vi "FullSetup.vi"() -> ()   [LabVIEW 2020]
uses:
  <vilib>/MakerHub/LINX/Private/Device/Type Defs/Stimulus Pulse.ctl
  <vilib>/MakerHub/LINX/Public/Peripherals/Analog/Analog Read 1 Chan.vi
  <vilib>/MakerHub/LINX/Public/Peripherals/Digital/Digital Write 1 Chan.vi
  <vilib>/MakerHub/LINX/Public/Peripherals/PWM/PWM Set Duty Cycle 1 Chan.vi
  <vilib>/MakerHub/LINX/Public/Peripherals/Analog/Analog Read N Chans.vi
  <vilib>/MakerHub/LINX/Public/Peripherals/Digital/Digital Write N Chans.vi
  <vilib>/MakerHub/LINX/Private/Local IO/LinxAnalogRead.vi
  <vilib>/MakerHub/LINX/Public/Utilities/Check Channel.vi
  <vilib>/MakerHub/LINX/Private/Local IO/LinxDigitalWrite.vi
  <vilib>/MakerHub/LINX/Public/Utilities/Open Serial.vi
  <vilib>/MakerHub/LINX/Private/Utilties/Generate Error.vi
  <vilib>/MakerHub/LINX/Public/Peripherals/PWM/PWM Set Duty Cycle N Chans.vi
  <vilib>/MakerHub/LINX/LMH-LINX.lvlib
  <vilib>/MakerHub/LINX/Private/Device/Device.lvlib
panel:
  out "Light Intensity":dbl
  out "Count Inside room":i32
  out "Distance OUT":dbl
  out "Waveform Chart 3":dbl(graph)
  in  "DO Channel OUT":u8
  in  "DI Channel OUT":u8
  out "Distance IN":dbl
  out "Waveform Chart":dbl(graph)
  in  "DO Channel IN":u8
  in  "DI Channe INl":u8
  in  "stop":bool
  out "Temperature":dbl
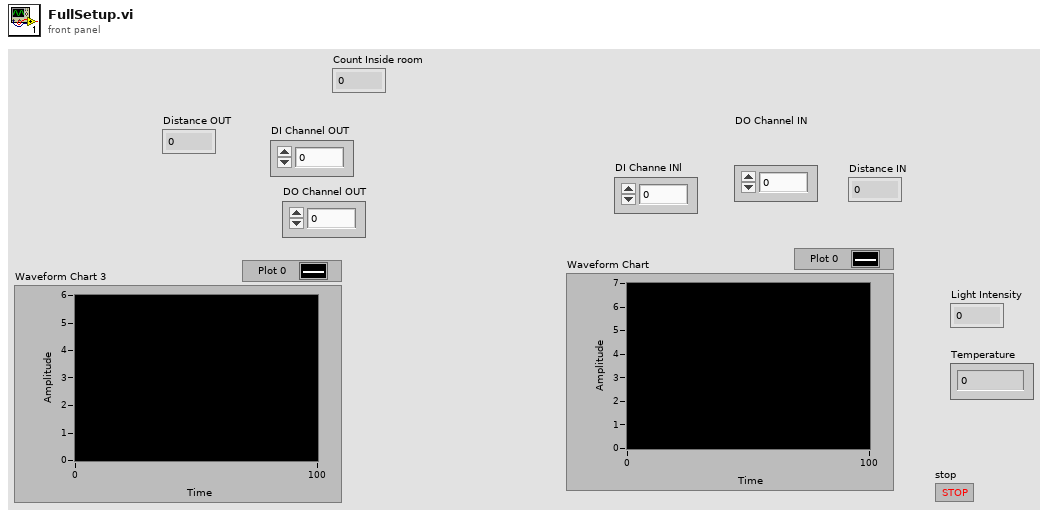
[diagram p1: front panel]
types:
  T1 = typedef "LMH-LINX.lvlib/LINX Ref.ctl" = cluster{"IO":T2, "Interface":T3, "LINX Device Config":T4}
  T2 = typedef "LMH-LINX.lvlib/Platform.ctl" = enum16{"Remote", "Local"}
  T3 = typedef "LMH-LINX.lvlib/Interface.ctl" = enum16{"Serial", "TCP"}
  T4 = typedef "LMH-LINX.lvlib/Device.lvlib/LINX Device Config.ctl" = cluster{"Interface":T3, "COM Port":refnum<visa-resource-name>, "TCP Configuration":T5, "Device Family":u8, "Device ID":u8, "Device Name":string, "TCP Ref":refnum<k5>, "Channels":T6}
  T5 = typedef "LMH-LINX.lvlib/Device.lvlib/TCP Config.ctl" = cluster{"IP Address":string, "Port":u16}
  T6 = typedef "LMH-LINX.lvlib/Channels.ctl" = cluster{"DI":u8[], "DO":u8[], "AI":u8[], "AO":u8[], "PWM":u8[], "QE":u8[], "UART":u8[], "I2C 2":u8[], "SPI":u8[], "CAN":u8[], "Servo":u8[], "AI Ref (V)":dbl, "AI Resolution (Bits)":u8, "AO Ref (V)":dbl, "AO Resolution (Bits)":u8}
  T7 = typedef "LMH-LINX.lvlib/Device.lvlib/Stimulus Pulse.ctl" = enum16{"None", "Active Low", "Active High"}
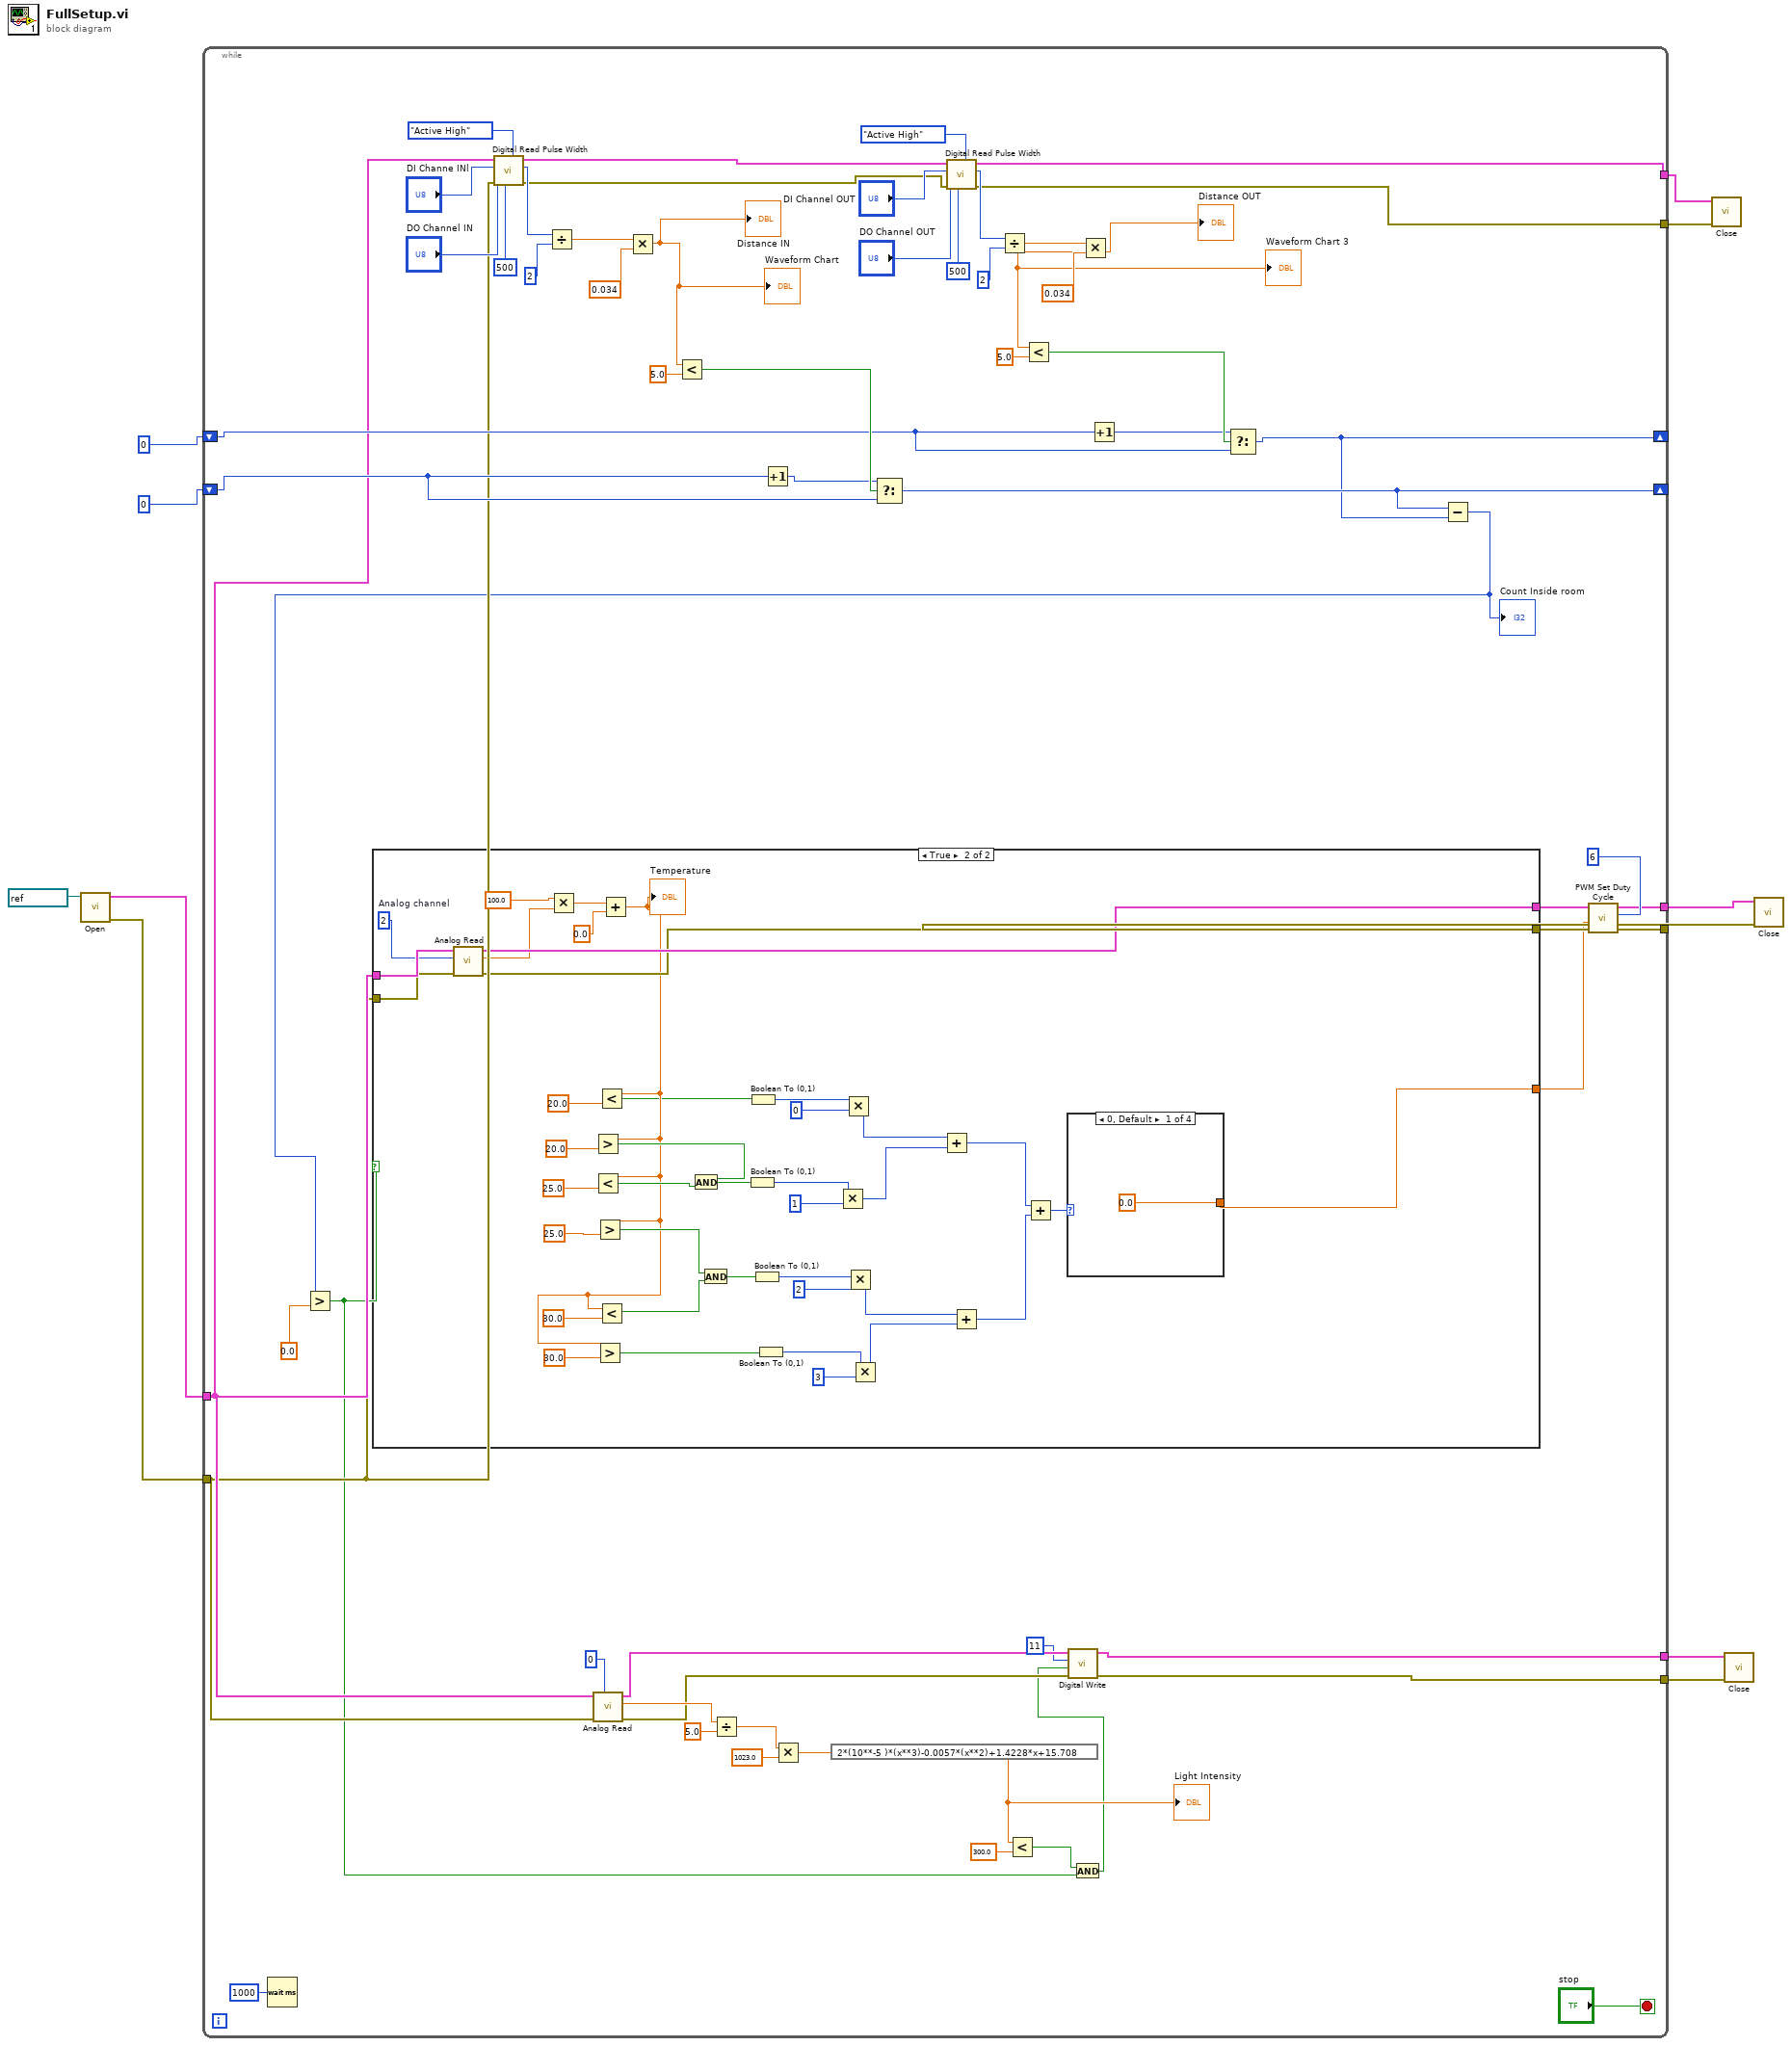
[diagram p0: block diagram]
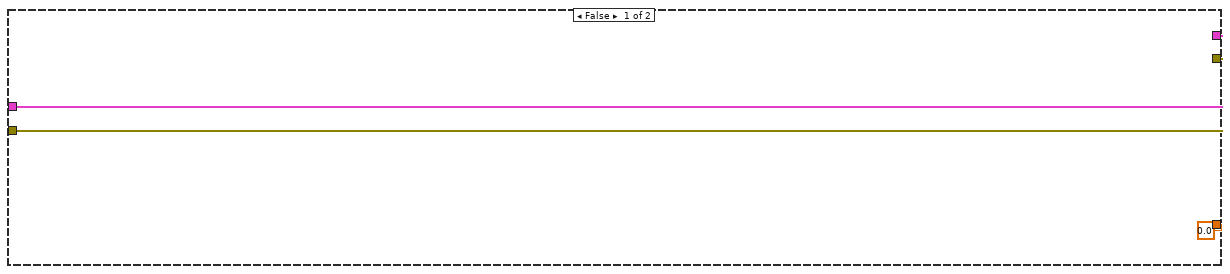
[diagram p2: hidden frame]
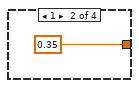
[diagram p3: hidden frame]
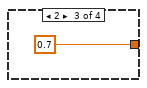
[diagram p4: hidden frame]
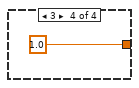
[diagram p5: hidden frame]
diagram:
  n1 = call-poly <vilib>:"Open.vi"("Serial Port"=refnum<visa-resource-name> "COM4") -> ("Error Out"=w9:errorcluster, "LINX Resource"=w11:T1)  [unwired: 8 in, 1 out]
  n2 = while {
    tunnel: w11 -> [w21]
    tunnel: [w66] -> w10
    tunnel: w9 -> [w20]
    tunnel: [w64] -> w8
    tunnel: [w38] -> w6
    shift-right: [w34] -> _
    shift-left: 0 -> [w37]
    shift-right: [w35] -> _
    shift-left: 0 -> [w36]
    tunnel: [w33] -> w3
    tunnel: [w18] -> w2
    tunnel: [w17] -> w1
    stop <- "stop" stop-if-true
    n3 = Wait (ms)(milliseconds to wait=u32 1000) -> ()  [unwired: 1 out]
    n4 = call <vilib>:"Digital Read Pulse Width.vi"("Stimulus Pulse (Active High)"=Stimulus_Pulse."Active High", "Timeout  (250 mS)"=u32 500, "Error In"=w20, "DO Channel"="DO Channel IN", "DI Channel"="DI Channe INl", "LINX Resource"=w21) -> ("Error Out"=w32:errorcluster, "Pulse Width (uS)"=w61:u32, "LINX Resource"=w47:T1)  [unwired: 3 in]
    n5 = Divide(x=w61, y=2) -> (x/y=w59:dbl)
    n6 = call-poly <vilib>:"Analog Read.vi"("Analog Ref Override (V)"=0, "Error In"=w20, "LINX Resource"=w21) -> ("Error Out"=w19:errorcluster, "Voltage"=w29:dbl, "LINX Resource"=w25:T1)  [unwired: 5 in, 1 out]
    n7 = Multiply(x=w59, y=0.034) -> (x*y=w46:dbl)
    "Waveform Chart" <- w46
    "Distance IN" <- w46
    n8 = Less?(x=w46, y=5.0) -> (x < y?=w42:bool)
    n9 = Divide(x=w29, y=5.0) -> (x/y=w27:dbl)
    n10 = Increment(x=w36) -> (x+1=w41:i32)
    n11 = Multiply(x=w27, y=1023.0) -> (x*y=w26:dbl)
    n12 = expression code="2*(10**-5 )*(x**3)-0.0057*(x**2)+1.4228*x+15.708"(w26) -> (w23:dbl)
    "Light Intensity" <- w23
    n13 = Select(t=w41, s=w42, f=w36) -> (s? t:f=w35:i32)
    n14 = call <vilib>:"Digital Read Pulse Width.vi"("Stimulus Pulse (Active High)"=Stimulus_Pulse."Active High", "Timeout  (250 mS)"=u32 500, "Error In"=w32, "DO Channel"="DO Channel OUT", "DI Channel"="DI Channel OUT", "LINX Resource"=w47) -> ("Error Out"=w33:errorcluster, "Pulse Width (uS)"=w53:u32, "LINX Resource"=w38:T1)  [unwired: 3 in]
    n15 = Divide(x=w53, y=2) -> (x/y=w51:dbl)
    n16 = Less?(x=w23, y=300.0) -> (x < y?=w15:bool)
    n17 = Multiply(x=w51, y=0.034) -> (x*y=w43:dbl)
    "Waveform Chart 3" <- w43
    "Distance OUT" <- w43
    n18 = Less?(x=w43, y=5.0) -> (x < y?=w40:bool)
    n19 = Increment(x=w37) -> (x+1=w39:i32)
    n20 = Select(t=w39, s=w40, f=w37) -> (s? t:f=w34:i32)
    n21 = Subtract(x=w35, y=w34) -> (x-y=w16:i32)
    "Count Inside room" <- w16
    n22 = Greater?(x=w16, y=0.0) -> (0:w13:bool)
    n23 = case shown="True" w13 {
      tunnel: w21 -> [w73 w114]
      tunnel: [w73 w113] -> w67
      tunnel: [w72 w112] -> w65
      tunnel: [0.0 w80] -> w70
      tunnel: w20 -> [w72 w75]
      frame False {
      }
      frame True {
        w111 = 2  # Analog channel
        n24 = call-poly <vilib>:"Analog Read.vi"("Error In"=w75, "Analog Channel"=w111, "LINX Resource"=w114) -> ("Error Out"=w112:errorcluster, "Voltage"=w109:dbl, "LINX Resource"=w113:T1)  [unwired: 5 in, 1 out]
        n25 = Multiply(x=100.0, y=w109) -> (x*y=w107:dbl)
        n26 = Add(x=w107, y=0.0) -> (x+y=w88:dbl)
        "Temperature" <- w88
        n27 = Greater?(x=w88, y=20.0) -> (0:w100:bool)
        n28 = Less?(x=w88, y=25.0) -> (x < y?=w99:bool)
        n29 = Greater?(x=w88, y=25.0) -> (0:w93:bool)
        n30 = Greater?(x=w88, y=30.0) -> (0:w76:bool)
        n31 = Less?(x=w88, y=20.0) -> (x < y?=w79:bool)
        n32 = Less?(x=w88, y=30.0) -> (x < y?=w92:bool)
        n33 = And(x=w100, y=w99) -> (x .and. y?=w78:bool)
        n34 = And(x=w93, y=w92) -> (x .and. y?=w77:bool)
        n35 = Boolean To (0,1)(Boolean=w78) -> (0, 1=w98:i16)
        n36 = Boolean To (0,1)(Boolean=w79) -> (0, 1=w105:i16)
        n37 = Boolean To (0,1)(Boolean=w77) -> (0, 1=w91:i16)
        n38 = Boolean To (0,1)(Boolean=w76) -> (0, 1=w86:i16)
        n39 = Multiply(x=w98, y=i16 1) -> (x*y=w96:i16)
        n40 = Multiply(x=w105, y=i16 0) -> (x*y=w103:i16)
        n41 = Multiply(x=w91, y=i16 2) -> (x*y=w89:i16)
        n42 = Multiply(x=w86, y=i16 3) -> (x*y=w84:i16)
        n43 = Add(x=w103, y=w96) -> (x+y=w83:i16)
        n44 = Add(x=w89, y=w84) -> (x+y=w82:i16)
        n45 = Add(x=w83, y=w82) -> (x+y=w81:i16)
        n46 = case shown="0, Default" w81 {
          tunnel: [0.0 0.35 0.7 1.0] -> w80
          frame 0, Default {
          }
          frame 1 {
          }
          frame 2 {
          }
          frame 3 {
          }
        }
      }
    }
    n47 = And(x=w15, y=w13) -> (x .and. y?=w14:bool)
    n48 = call-poly <vilib>:"Digital Write.vi"("Error In"=w19, "Output Value"=w14, "DO Channel"=u8 11, "LINX Resource"=w25) -> ("Error Out"=w17:errorcluster, "LINX Resource"=w18:T1)  [unwired: 6 in]
    n49 = call-poly <vilib>:"PWM Set Duty Cycle.vi"("Error In"=w65, "Duty Cycle (0-1)"=w70, "PWM Channel"=u8 6, "LINX Resource"=w67) -> ("Error Out"=w64:errorcluster, "LINX Resource"=w66:T1)  [unwired: 6 in]
  }
  n50 = call <vilib>:"Close.vi"("Error In"=w3, "LINX Resource"=w6) -> ()  [unwired: 9 in, 1 out]
  n51 = call <vilib>:"Close.vi"("Error In"=w1, "LINX Resource"=w2) -> ()  [unwired: 9 in, 1 out]
  n52 = call <vilib>:"Close.vi"("Error In"=w8, "LINX Resource"=w10) -> ()  [unwired: 9 in, 1 out]
